vi "Read CDO.vi"(8 "error in (no error)":errorcluster, 11 "SD Module in":refnum<class "SD Module.lvclass">) -> (0 "error out":errorcluster, 2 "CDO":T1, 3 "SD Module out":refnum<class "SD Module.lvclass">)   [LabVIEW 2017, in "Modules.lvlib" / "SD Module.lvclass"]
uses:
  SD Module.lvclass
  Type Defs/CDO.ctl
  Type Defs/CDO Channel.ctl
  SD Module.lvclass/SD Module.ctl
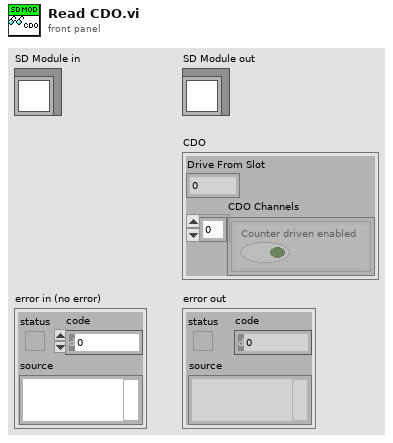
[diagram p1: front panel]
types:
  T1 = typedef "Modules.lvlib/SD Module.lvclass/CDO.ctl" = cluster{"Drive From Slot":u32, "CDO Channels":T2[]}
  T2 = typedef "Modules.lvlib/SD Module.lvclass/CDO Channel.ctl" = cluster{"Counter driven enabled":bool}
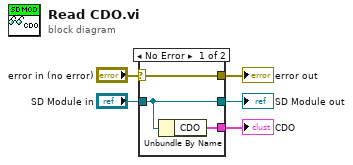
[diagram p0: block diagram]
diagram:
  n1 = case shown="No Error" "error in (no error)" {
    selector: "error in (no error)" -> [w8 w9]
    tunnel: [w8 w9] -> w4
    tunnel: [w7 w10] -> w2
    tunnel: "SD Module in" -> [w7 w10]
    tunnel: [w6 _] -> w1
    frame No Error {
      n2 = Unbundle By Name(w7) -> ("CDO"=w6:T1)
    }
    frame Error {
    }
  }
  "error out" <- w4
  "SD Module out" <- w2
  "CDO" <- w1
